vi "formal - Copy.vi"() -> ()   [LabVIEW 2011]
uses:
  <vilib>/DAQmx/read.llb/DAQmx Read (Analog 1D Wfm NChan NSamp).vi
  <vilib>/DAQmx/configure/timing.llb/DAQmx Timing (Sample Clock).vi
  <vilib>/DAQmx/miscellaneous.llb/DAQmx Fill In Error Info.vi
  C:/Program Files (x86)/National Instruments/LabVIEW 2011/resource/objmgr/daqmx.rc
panel:
  in  "stop":bool
  in  "Tab Control":T1(tab)
  out "Utility Usage Array":cluster{bool, string}[][](array[cluster])=[[{TRUE, "hjk"}, {FALSE, ""}, {FALSE, ""}, {FALSE, ""}], [{TRUE, "hjk"}, {FALSE, ""}, {FALSE, ""}, {FALSE, ""}], [{FALSE, ""}, {FALSE, ""}, {FALSE, ""}, {FALSE, ""}], [{FALSE, ""}, {FALSE, ""}, {FALSE, ""}, {FALSE, ""}], [{FALSE, ""}, {FALSE, ""}, {FALSE, ""}, {FALSE, ""}], [{FALSE, ""}, {FALSE, ""}, {FALSE, ""}, {FALSE, ""}], [{FALSE, ""}, {FALSE, ""}, {FALSE, ""}, {FALSE, ""}], [{FALSE, ""}, {FALSE, ""}, {FALSE, ""}, {FALSE, ""}]]
  in  "SXCI Chassis Name":string="/SC1"
  in  "file path":path=path "M:/github/DAQP/xml_temp.xml"
  in  "task out":refnum<k21>="new Task"
  in  "error in":errorcluster
  in  "custom scale name":tag="linear1"
  in  "voltage excitation source":i32(ring)=10200 items=["Internal"=10200, "External"=10167, "None"=10230]
  in  "error out":errorcluster
  in  "sample rate":dbl=1000.0
  in  "number of samples per channel (buffer size)":i32=10000000
  in  "number of samples per channel":i32=100
  out "data":waveform(dbl)[](array[waveform])=[{"t0"=timestamp(3441485051.542661 s since 1904-01-01), "dt"=0.001, "Y"=[0.1172447484123107, 0.07327796775769418, -0.048851978505129456, 0.09281875915974597, -0.04396678065461651, -0.21006350757205666, 0.3224230581338544, -0.21983390327308255, -0.19540791402051783, 0.18563751831949193, 0.28334147532975085, 0.1074743527112848, -0.17586712261846604, 0.03419638495359062, 0.04396678065461651, -0.2247191011235955, 0.2247191011235955, -0.13678553981436248, 0.29311187103077674, 0.3517342452369321, 0.09281875915974597, -0.2149487054225696, -0.1612115290669272, -0.039081582804103565, 0.13190034196384953, 0.13190034196384953, 0.2882266731802638, -0.029311187103077674, 0.13190034196384953, 0.3419638495359062, -0.04396678065461651, 0.28334147532975085, -0.0635075720566683, 0.08304836345872008, 0.12212994626282364, 0.13678553981436248, 0.18563751831949193, -0.16609672691744015, 0.361504640937958, -0.15632633121641426, 0.03419638495359062, 0.180752320468979, 0.15144113336590131, 0.004885197850512946, 0.3419638495359062, -0.019540791402051783, 0.21983390327308255, 0.19540791402051783, -0.2344894968246214, -0.10258915486077186, -0.14655593551538837, 0.23937469467513434, 0.12212994626282364, 0.03419638495359062, -0.14655593551538837, 0.09770395701025891, 0.07816316560820713, -0.039081582804103565, 0.1270151441133366, 0.3126526624328285, 0.004885197850512946, 0.10258915486077186, -0.20517830972154372, 0.18563751831949193, 0.2540302882266732, 0.15632633121641426, 0.2589154860771861, -0.20029311187103077, -0.048851978505129456, 0.0635075720566683, -0.13190034196384953, 0.2247191011235955, 0.13678553981436248, -0.08793356130923302, -0.21006350757205666, 0.004885197850512946, -0.11235955056179775, 0.009770395701025891, 0.21006350757205666, -0.21983390327308255, -0.029311187103077674, -0.13190034196384953, -0.17586712261846604, 0.0, 0.20517830972154372, -0.10258915486077186, -0.08304836345872008, -0.18563751831949193, -0.20517830972154372, 0.18563751831949193, 0.2344894968246214, 0.23937469467513434, -0.048851978505129456, 0.20029311187103077, -0.03419638495359062, -0.13190034196384953, 0.0537371763556424, -0.1172447484123107, -0.05862237420615535, -0.07816316560820713], "attributes"=variant("NI_ChannelName"=variant(string "hjk"))}]
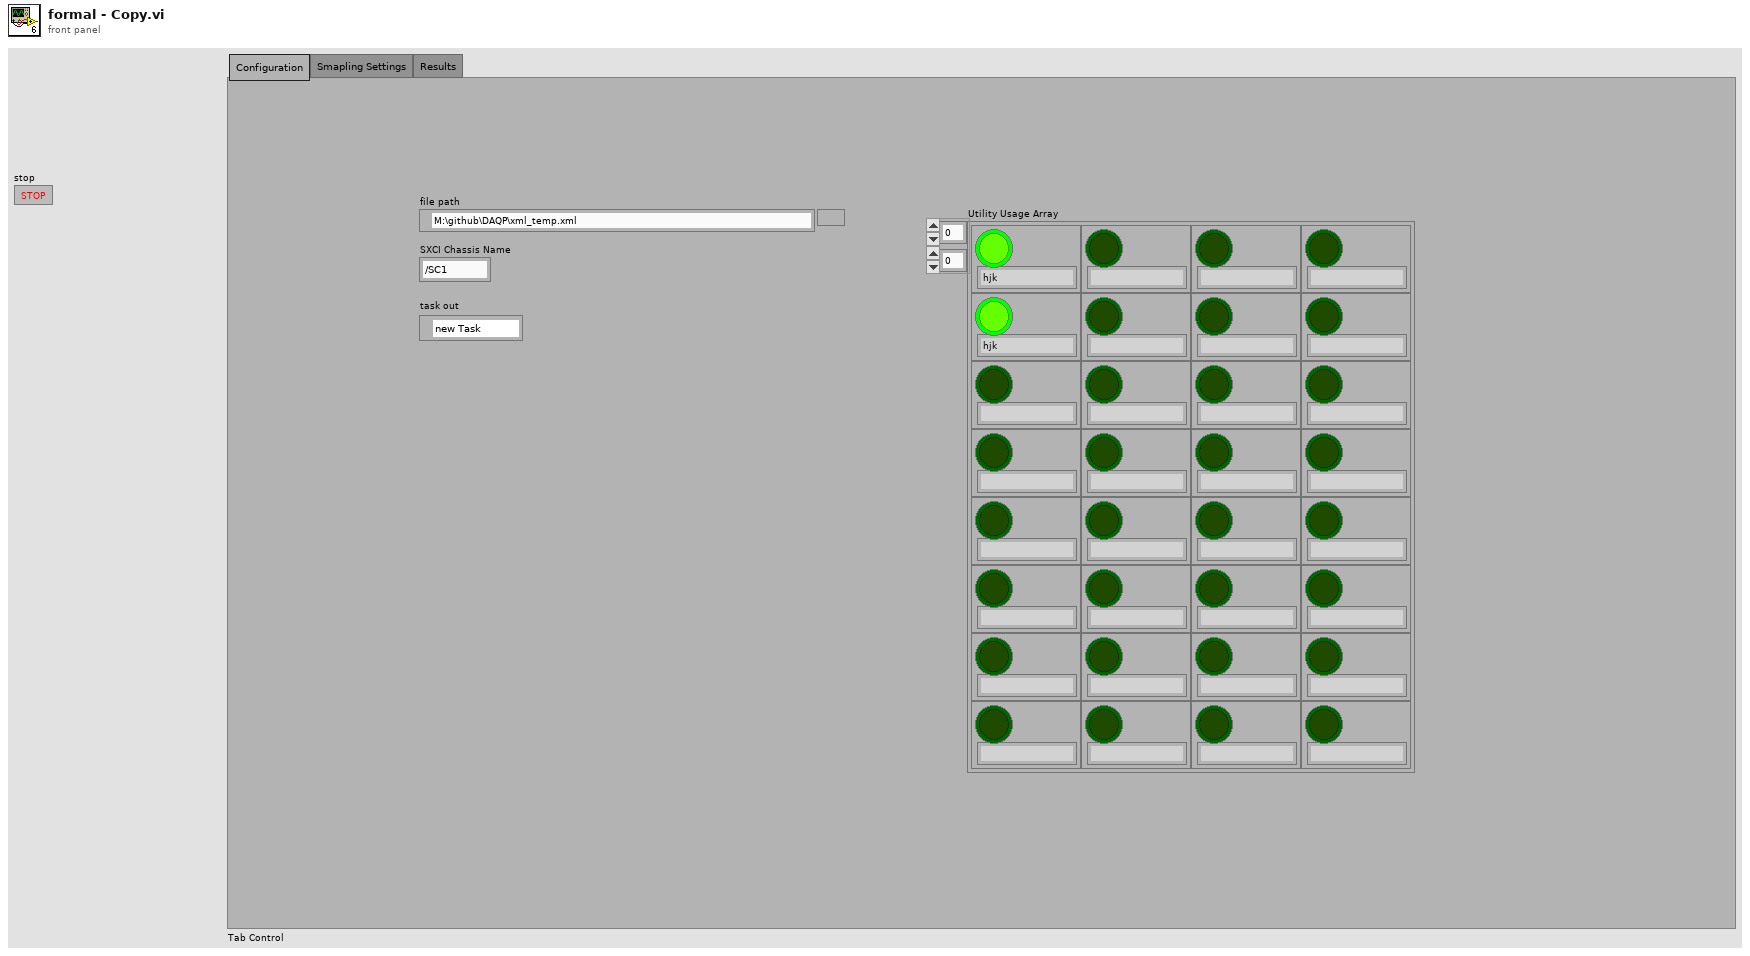
[diagram p1: front panel]
types:
  T1 = enum32{"Configuration", "Smapling Settings", "Results"}
  T2 = cluster{string[], "Voltage_cluster":cluster{dbl, dbl, dbl, dbl, bool, dbl, dbl}, "Strain_cluster":cluster{dbl, dbl, dbl, dbl, bool, dbl, dbl, dbl, dbl, string}}[]
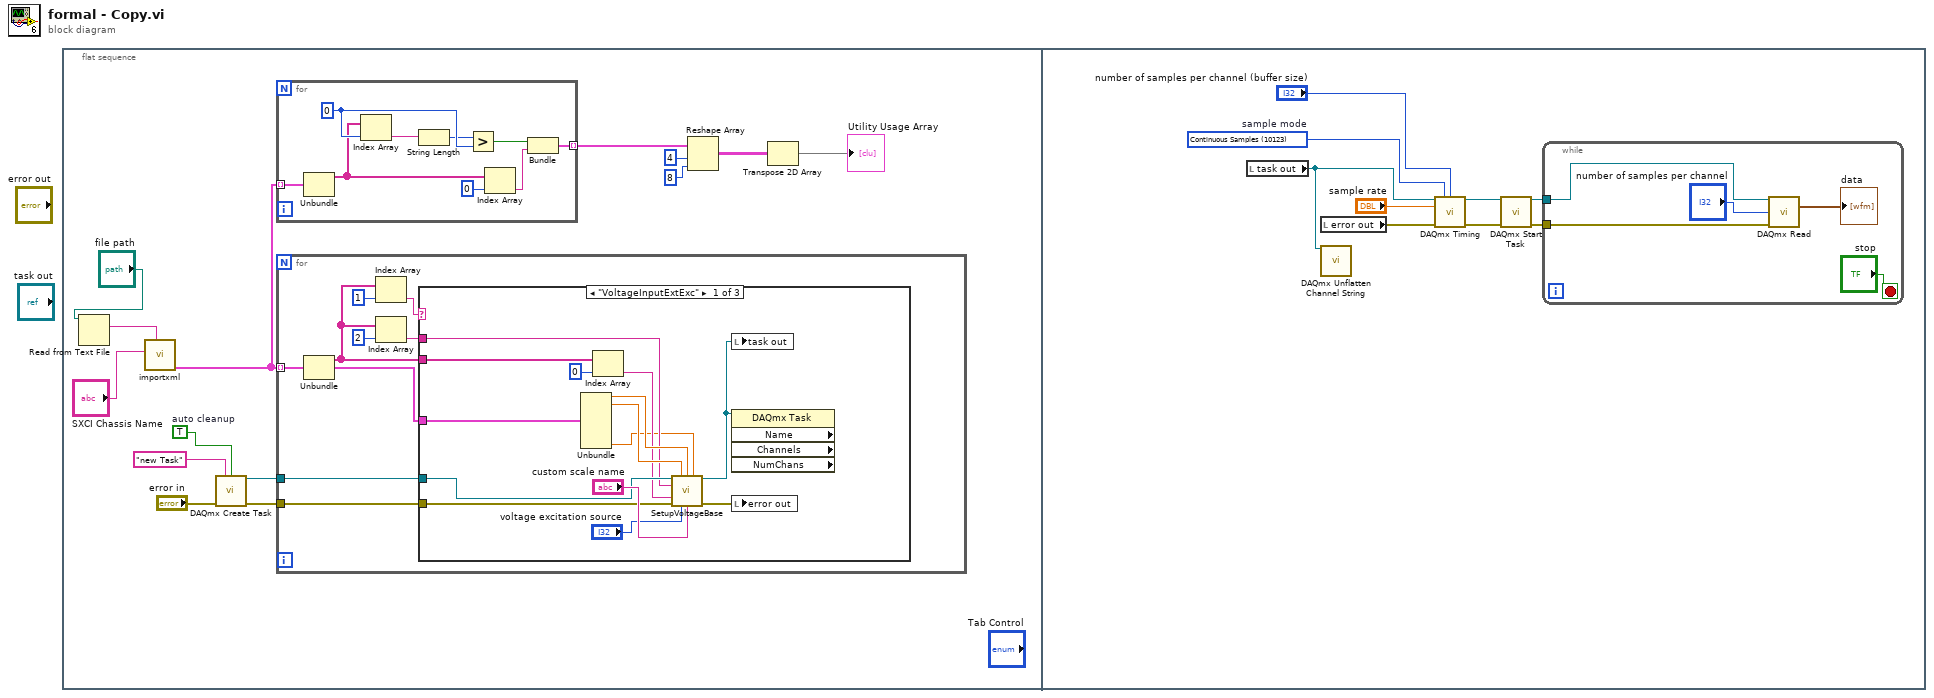
[diagram p0: block diagram]
diagram:
  n1 = flat-sequence {
    frame #0 {
      w4 = TRUE  # auto cleanup
      n2 = Read from Text File(file (use dialog)="file path") -> (text=w13:string)  [unwired: 3 in, 3 out]
      n3 = call "importxml.vi"("String"=w13, "sc"="SXCI Chassis Name") -> ("output array"=w2:T2)  [unwired: 9 in]
      n4 = call <vilib>:"DAQmx Create Task.vi"("new task name"="new Task", "auto cleanup"=w4, "error in"="error in") -> ("task out"=w6:refnum<k21>, "error out"=w5:errorcluster)  [unwired: 2 in, 9 out]
      n5 = for {
        tunnel: w2 -> [w46] mode=indexing
        tunnel: [w38] -> w8 mode=indexing
        w44 = 0 ("index")
        n6 = Unbundle(w46) -> (w41:string[])  [unwired: 2 out]
        n7 = Index Array(array=w41, index=w44) -> (element=w45:string)
        n8 = String Length(string=w45) -> (length=w43:i32)
        n9 = Greater?(x=w43, y=w44) -> (0:w40:bool)
        n10 = Index Array(array=w41, index=0) -> (element=w39:string)
        n11 = Bundle(w40, w39) -> (w38:cluster{bool, string})  [unwired: 1 in]
      }
      n12 = for {
        tunnel: w2 -> [w23] mode=indexing
        tunnel: w6 -> [w20]
        tunnel: w5 -> [w19]
        n13 = Unbundle(w23) -> (w16:string[], "Voltage_cluster"=w18:cluster{dbl, dbl, dbl, dbl, bool, dbl, dbl})  [unwired: 1 out]
        n14 = Index Array(array=w16, index=1) -> (element=w21:string)
        n15 = Index Array(array=w16, index=2) -> (element=w15:string)
        n16 = case shown="\"VoltageInputExtExc\"" w21 {
          tunnel: w20 -> [w33 _ _]
          tunnel: w19 -> [w32 _ _]
          tunnel: w18 -> [w31 _ _]
          tunnel: w16 -> [w30 _ _]
          tunnel: w15 -> [w26 _ _]
          frame "VoltageInputExtExc" {
            n17 = Unbundle(w31) -> (w36:dbl, w35:dbl, w24:dbl)  [unwired: 4 out]
            n18 = Index Array(array=w30, index=0) -> (element=w28:string)
            n19 = call "SetupVoltageBase.vi"("Refnum in"=w33, "Numeric"=w35, "Numeric 2"=w36, "excitation value"=w24, "physical channel"=w26, "String"=w28, "error in (no error)"=w32, "voltage excitation source"="voltage excitation source", "custom scale name"="custom scale name") -> ("Refnum out"=w25:refnum<k21>, "error out"=w27:errorcluster)  [unwired: 5 in]
            n20 = local write "task out"(w25) -> ()
            n21 = property class="DAQmx Task" props=["Name", "Channels", "NumChans"](reference=w25) -> ()  [unwired: 1 in, 5 out]
            n22 = local write "error out"(w27) -> ()
          }
          frame "Null", Default {
          }
          frame "VoltageInputIntExc" {
          }
        }
      }
      n23 = Reshape Array(w8, 4 ("dimension size"), 8 ("dimension size")) -> (w10:cluster{bool, string}[][])
      n24 = Transpose 2D Array(2D array=w10) -> (transposed array=→"Utility Usage Array":cluster{bool, string}[][])
    }
    frame #1 {
      w53 = 10123 items=["Finite Samples"=10178, "Continuous Samples"=10123, "Hardware Timed Single Point"=12522]  # sample mode
      n25 = local read "task out"() -> (w50:refnum<k21>)
      n26 = local read "error out"() -> (w49:errorcluster)
      n27 = call <vilib>:"DAQmx Unflatten Channel String.vi"("names in"=w50) -> ()  [unwired: 1 in, 14 out]
      n28 = call-poly <vilib>:"DAQmx Timing.vi"("task/channels in"=w50, "sample mode"=w53, "samples per channel"="number of samples per channel (buffer size)", "rate"="sample rate", "error in"=w49) -> ("task out"=w52:refnum<k21>, "error out"=w51:errorcluster)  [unwired: 2 in, 7 out]
      n29 = call <vilib>:"DAQmx Start Task.vi"("task/channels in"=w52, "error in"=w51) -> ("task out"=w48:refnum<k21>, "error out"=w47:errorcluster)  [unwired: 12 out]
      n30 = while {
        tunnel: w48 -> [w60]
        tunnel: w47 -> [w59]
        stop <- "stop" stop-if-true
        n31 = call-poly <vilib>:"DAQmx Read.vi"("task/channels in"=w60, "number of samples per channel"="number of samples per channel", "error in"=w59) -> ("data"=→"data":waveform(dbl)[])  [unwired: 10 in, 2 out]
      }
    }
  }
